vi "2s Compliment To Decimal.vi"(4 "Bit Width (8)":i32=8, 5 "2s Comp Number":u16) -> (1 "Decimal Number":i32)   [LabVIEW 2020, in "LMH-Toolbox.lvlib"]
doc: "Convert the given 2's compliment number to decimal. The width field specifies the number of bits in the 2's compliment number."
uses:
  LMH-Toolbox.lvlib
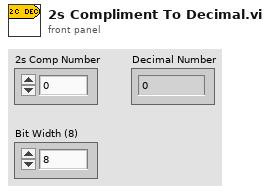
[diagram p1: front panel]
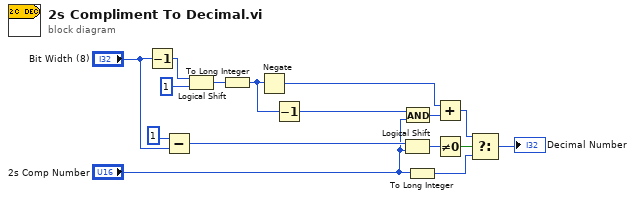
[diagram p0: block diagram]
diagram:
  n1 = Decrement(x="Bit Width (8)") -> (x-1=w11:i32)
  n2 = Subtract(x=1, y="Bit Width (8)") -> (x-y=w6:i32)
  n3 = Logical Shift(y=w11, x=u32 1) -> (x << y=w10:u32)
  n4 = To Long Integer(number=w10) -> (32bit integer=w5:i32)
  n5 = Negate(x=w5) -> (-x=w9:i32)
  n6 = Decrement(x=w5) -> (x-1=w4:i32)
  n7 = Logical Shift(y=w6, x="2s Comp Number") -> (x << y=w16:u16)
  n8 = And(x=w4, y="2s Comp Number") -> (x .and. y?=w14:i32)
  n9 = To Long Integer(number="2s Comp Number") -> (32bit integer=w2:i32)
  n10 = Add(x=w9, y=w14) -> (x+y=w13:i32)
  n11 = Not Equal To 0?(x=w16) -> (x != 0?=w15:bool)
  n12 = Select(t=w13, s=w15, f=w2) -> (s? t:f=→"Decimal Number":i32)
